vi "IndoorData_CleanUp.vi"(5 "error in (no error)":errorcluster) -> (19 "error out":errorcluster)   [LabVIEW 2014, in "IndoorData.lvclass"]
uses:
  IndoorData.lvclass
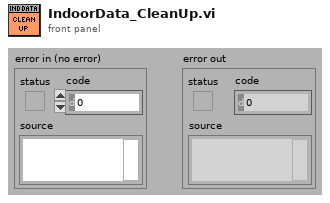
[diagram p1: front panel]
types:
  T1 = typedef "IndoorData.lvclass/ObjectAttributes.ctl" = cluster{"DebugData":T2}
  T2 = typedef "IndoorData.lvclass/DebugData.ctl" = cluster{"Rev":string, "Location":string, "LoopIdx":i32, "PiCoreTemp":dbl, "Error":errorcluster}
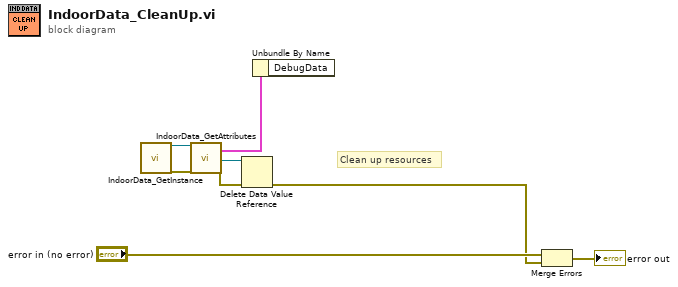
[diagram p0: block diagram]
diagram:
  # "Clean up resources"
  n1 = call "IndoorData_GetInstance.vi"() -> ("reference out"=w5:refnum<class "IndoorData.lvclass">, "error out"=w6:errorcluster)  [unwired: 15 in, 3 out]
  n2 = call "IndoorData_GetAttributes.vi"("reference in"=w5, "error in (no error)"=w6) -> ("Data"=w7:T1, "DataRef"=w3:refnum<data-value>, "error out"=w4:errorcluster)  [unwired: 14 in, 1 out]
  n3 = Delete Data Value Reference(data value reference=w3, error in=w4) -> (error out=w1:errorcluster)  [unwired: 1 out]
  n4 = Unbundle By Name(w7) -> ()  [unwired: 1 out]
  n5 = Merge Errors("error in (no error)", w1) -> (→"error out":errorcluster)
